vi "Write_image_csv.vi"(9 "Image Pixels (U16)":u16[][](array[numeric]), 10 "Chose where to save the files":enum32{"C", "U"}(ring), 11 "seconds\n between acquistions":u32) -> ()   [LabVIEW 2023]
uses:
  <vilib>/Utility/file.llb/Write Delimited Spreadsheet (I64).vi
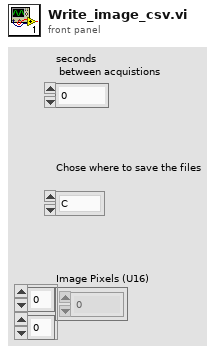
[diagram p1: front panel]
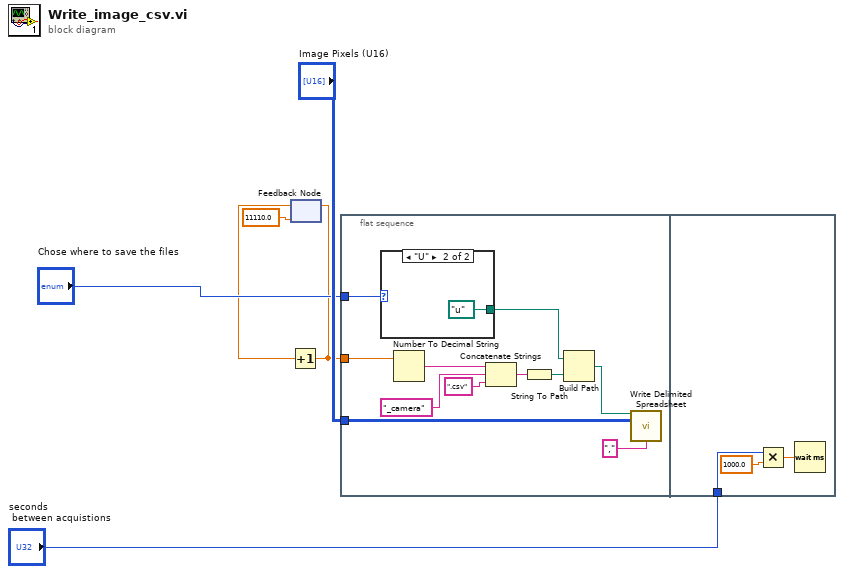
[diagram p0: block diagram]
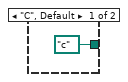
[diagram p2: hidden frame]
diagram:
  n1 = feedback #1(11110.0) -> (w3:dbl)
  n2 = Increment(x=w3) -> (x+1=w2:dbl)
  n3 = feedback-in #1(w2) -> ()
  n4 = flat-sequence {
    tunnel: w2 -> [w13]
    tunnel: "Image Pixels (U16)" -> [w9]
    tunnel: "Chose where to save the files" -> [w7]
    tunnel: "seconds\n between acquistions" -> [w20]
    frame #0 {
      n5 = case shown="\"U\"" w7 {
        tunnel: [path "c:/" path "u:/"] -> w8
        frame "C", Default {
        }
        frame "U" {
        }
      }
      n6 = Number To Decimal String(number=w13) -> (decimal integer string=w16:string)  [unwired: 1 in]
      n7 = Concatenate Strings(w16, "_camera" ("string"), ".csv" ("string")) -> (w17:string)
      n8 = String To Path(string=w17) -> (path=w15:path)
      n9 = Build Path(base path=w8, name or relative path=w15) -> (appended path=w14:path)
      n10 = call-poly <vilib>:"Write Delimited Spreadsheet.vi"("file path (dialog if empty)"=w14, "2D data"=w9, "delimiter (\\t)"="," ("delimiter (\\t)")) -> ()  [unwired: 11 in, 2 out]
    }
    frame #1 {
      n11 = Multiply(x=w20, y=1000.0) -> (x*y=w21:dbl)
      n12 = Wait (ms)(milliseconds to wait=w21) -> ()  [unwired: 1 out]
    }
  }
